vi "VI Folder Action Template.vi"(6 "Exclude Pattern":string, 8 "error in (no error)":errorcluster, 11 "VI Folder":path) -> (0 "error out":errorcluster, 3 "VI List":path[](array[path]))   [LabVIEW 2016, in "SLL Scripting.lvlib"]
doc: "This template VI is useful to quickly code any action that needs to be done to all VIs in a folder."
uses:
  SLL Scripting.lvlib
  <vilib>/regexp/Match Regular Expression.xnode
panel:
  out "Progress":i32
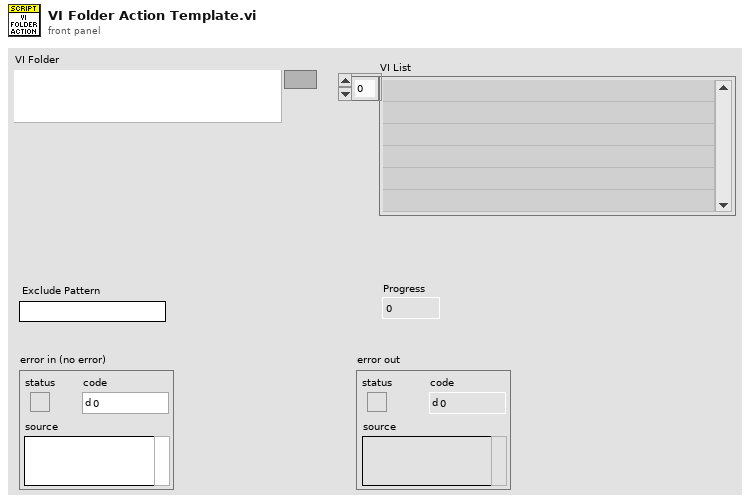
[diagram p1: front panel]
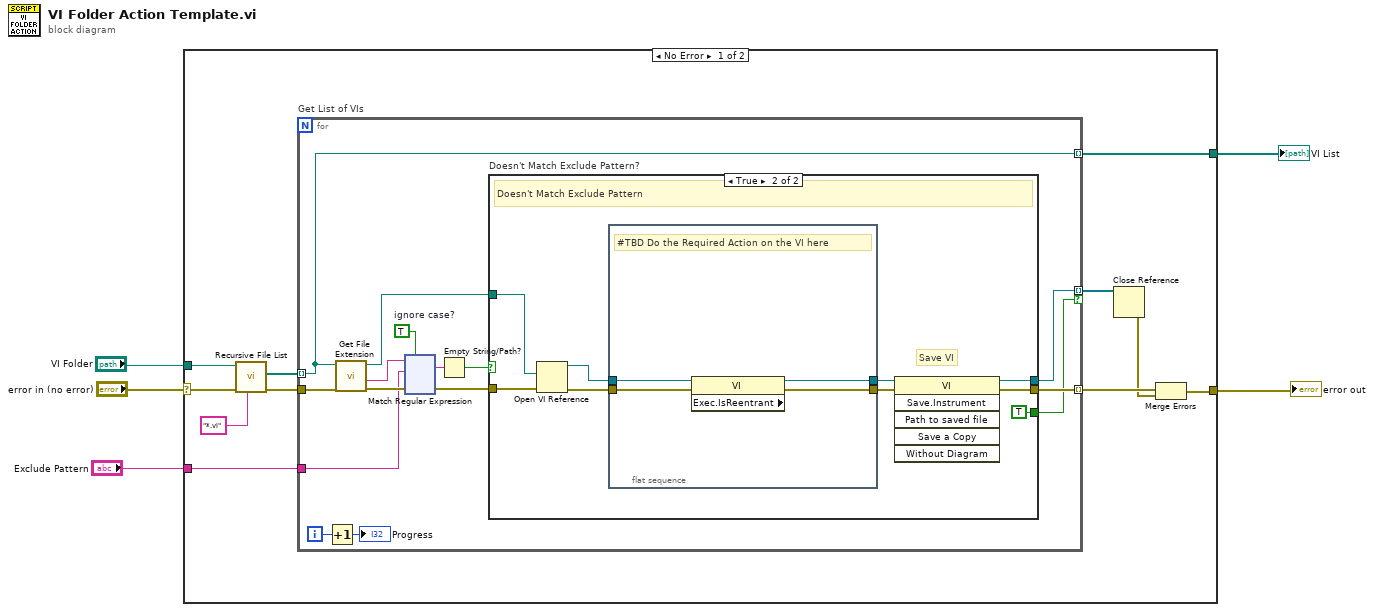
[diagram p0: block diagram]
diagram:
  n1 = case shown="No Error" "error in (no error)" {
    selector: "error in (no error)" -> [w11 w160]
    tunnel: "VI Folder" -> [w15 _]
    tunnel: [w12 _] -> w4
    tunnel: [w7 w160] -> w2
    tunnel: "Exclude Pattern" -> [w6 _]
    frame No Error {
      n2 = call <vilib>:"Recursive File List.vi"("pattern"="*.vi", "error in (no error)"=w11, "Folder Path"=w15) -> ("error out"=w10:errorcluster, "All Files in Dir"=w13:path[])  [unwired: 4 in, 3 out]
      n3 = for "Get List of VIs" {
        tunnel: [w29] -> w16 mode=indexing if=w20
        tunnel: w13 -> [w18] mode=indexing
        tunnel: [w18] -> w12 mode=indexing
        tunnel: w10 -> [w24]
        tunnel: [w30] -> w9 mode=indexing
        tunnel: w6 -> [w19]
        i -> [w31]
        w27 = TRUE  # ignore case?
        n4 = Increment(x=w31) -> (x+1=→"Progress":i32)
        n5 = call <vilib>:"Get File Extension.vi"("error in (no error)"=w24, "file"=w18) -> ("error out"=w28:errorcluster, "filename without extension"=w26:string, "dup file"=w21:path)  [unwired: 5 in, 2 out]
        n6 = xnode "Match Regular Expression"("input string"=w26, "regular expression"=w19, "error in"=w28, "ignore case? (F)"=w27) -> ("whole match"=w25:string, "error out"=w23:errorcluster)  [unwired: 2 in, 3 out]
        n7 = Empty String/Path?(string/path=w25) -> (empty?=w22:bool)
        n8 = case "Doesn't Match Exclude Pattern?" shown="True" w22 {
          tunnel: [w32 w38] -> w30
          tunnel: [_ w36] -> w29
          tunnel: w23 -> [w32 w35]
          tunnel: w21 -> [_ w34]
          tunnel: [_ TRUE] -> w20
          frame False {
            # "Matches Exclude Pattern, Skip."
          }
          frame True {
            # "Save VI"
            # "Doesn't Match Exclude Pattern"
            n9 = Open VI Reference(vi path=w34, error in (no error)=w35) -> (vi reference=w41:refnum<vi>, error out=w40:errorcluster)  [unwired: 4 in]
            n10 = flat-sequence {
              tunnel: w41 -> [w43]
              tunnel: w40 -> [w45]
              tunnel: [w44] -> w39
              tunnel: [w42] -> w37
              frame #0 {
                # "#TBD Do the Required Action on the VI here"
                n11 = property class="VI" props=["Exec.IsReentrant"](reference=w43, error in=w45) -> (reference out=w42:refnum<vi>, error out=w44:errorcluster)  [unwired: 1 out]
              }
            }
            n12 = invoke class="VI" method="Save.Instrument"(reference=w37, error in=w39) -> (reference out=w36:refnum<vi>, error out=w38:errorcluster)  [unwired: 4 in, 4 out]
          }
        }
      }
      n13 = Close Reference(reference=w16) -> (error out=w8:errorcluster)  [unwired: 1 in]
      n14 = Merge Errors(w9, w8) -> (w7:errorcluster)
    }
    frame Error {
    }
  }
  "error out" <- w2
  "VI List" <- w4
